vi "Timer_Close.vi"(8 "error in (no error)":errorcluster, 11 "Timer Data Reference (in)":refnum<data-value>) -> (0 "error out":errorcluster)   [LabVIEW 2024]
doc: "Closes Timer DVR\n--------\nPaulo Rossi\nprossi@aurumautomation.ca\n©2024 Aurum Automation Inc.\nOpen-Sourced per GNU GPL v3\n\nYou should have received a copy of the GNU General Public License along with this program. If not, see <https://www.gnu.org/licenses/>."
uses:
  Timer_Data.ctl
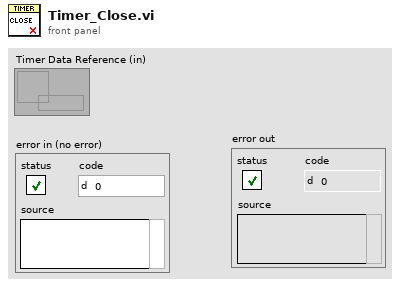
[diagram p1: front panel]
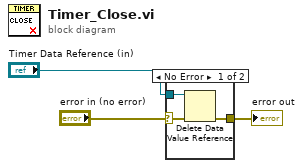
[diagram p0: block diagram]
diagram:
  n1 = case shown="No Error" "error in (no error)" {
    selector: "error in (no error)" -> [w6 w7]
    tunnel: [w5 w7] -> w2
    tunnel: "Timer Data Reference (in)" -> [w4 _]
    frame No Error {
      n2 = Delete Data Value Reference(data value reference=w4, error in=w6) -> (error out=w5:errorcluster)  [unwired: 1 out]
    }
    frame Error {
    }
  }
  "error out" <- w2
